vi "Fit Plots Cluster to Array.vi"(0 "Fit Plots in":T2, 1 "Plot Interpolation":T1=enum."Line (-)", 2 "Decay Fit Plot Name":string, 3 "Color Array in":u32[](array[colorbox])) -> (5 "Residuals Plot?":bool, 6 "Fit Plot Array":cluster{"t Array":dbl[], "Fitted Array":dbl[]}[](array[cluster]), 7 "Plot Names":string[](array[string]), 8 "CI Plots?":bool, 9 "Color Array out":u32[](array[colorbox]))   [LabVIEW 2021, in "AlliGator Decay Fit.lvlib"]
uses:
  AlliGator/Decay Analysis/Decay Fit/AlliGator Decay Fit.lvlib
  Fit Plots.ctl
  Graphs/LabVIEW Plot Interpolation.ctl
  Graphs/XY Graph/XY Graph Add-Ons.lvlib
  Graphs/Graphs.lvlib
  Fits.lvlib
panel:
  # "see the License on the block diagram (Ctrl+E or Window:Show Block Diagram)"
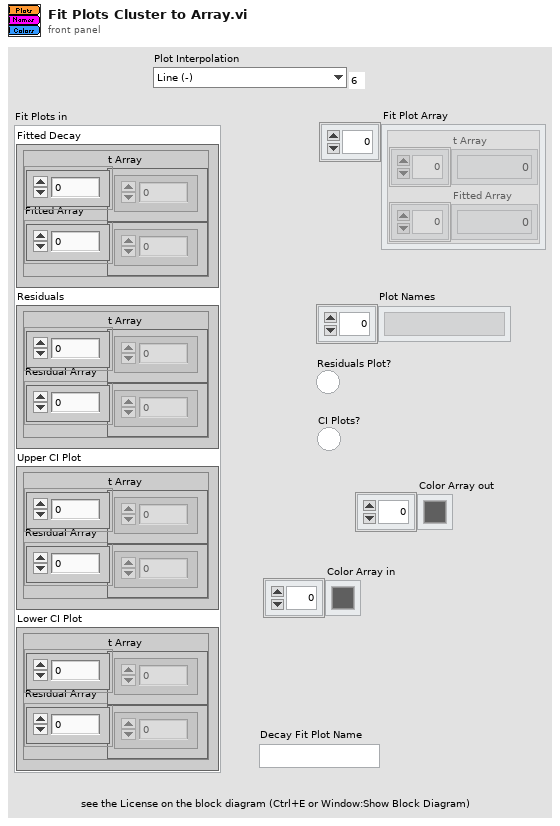
[diagram p1: front panel]
types:
  T1 = typedef "Graphs.lvlib/LabVIEW Plot Interpolation.ctl" = enum16{"Point (.)", "Stepwise Right (--.)", "Line + Point (\\. /)", "Stepwise Left (.--)", "Stepwise Centered (-.-)", "Stepwise Vertical (|.|)", "Line (-)", "Use Previous Plot's Style"}
  T2 = typedef "Fits.lvlib/Fit Plots.ctl" = cluster{"Fitted Decay":cluster{"t Array":dbl[], "Fitted Array":dbl[]}, "Residuals":cluster{"t Array":dbl[], "Residual Array":dbl[]}, "Upper CI Plot":cluster{"t Array":dbl[], "Residual Array":dbl[]}, "Lower CI Plot":cluster{"t Array":dbl[], "Residual Array":dbl[]}}
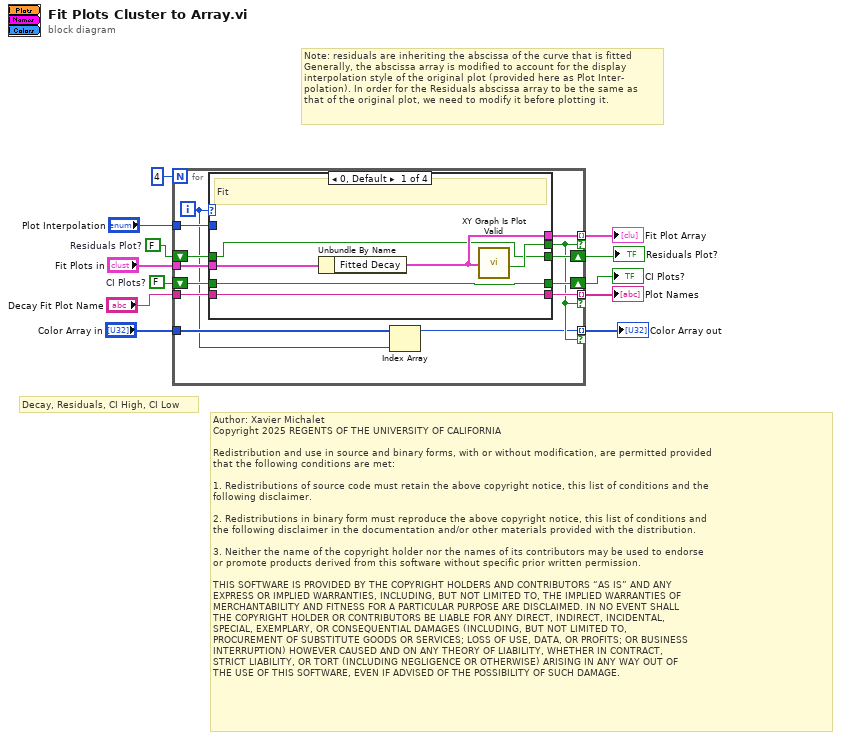
[diagram p0: block diagram]
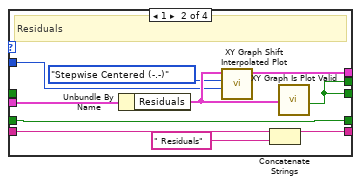
[diagram p2: hidden frame]
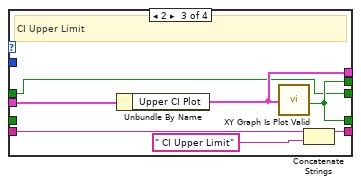
[diagram p3: hidden frame]
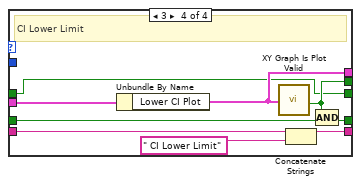
[diagram p4: hidden frame]
diagram:
  w3 = FALSE  # Residuals Plot?
  w7 = FALSE  # CI Plots?
  # "Decay, Residuals, CI High, CI Low"
  # "Note: residuals are inheriting the abscissa of the curve that is fitted\nGenerally, the abscissa array is modified to account for the display\ninterpolation style of the original plot (provided here as Plot Inter-\npolation). In order for the Residuals abscissa array to be the same as\nthat of the original plot, we need to modify it before plotting it."
  # "Author: Xavier Michalet\nCopyright 2025 REGENTS OF THE UNIVERSITY OF CALIFORNIA\n\nRedistribution and use in source and binary forms, with or without modification, are permitted provided\nthat the following conditions are met:\n\n1. Redistributions of source code must retain the above copyright notice, this list of conditions and the\nfollowing disclaimer.\n\n2. Redistributions in binary form must reproduce the above copyright notice, this list of conditions and\nthe following disclaimer in the documentation and/or other materials provided with the distribution.\n\n3. Neither the name of the copyright holder nor the names of its contributors may be used to endorse \nor promote products derived from this software without specific prior written permission.\n\nTHIS SOFTWARE IS PROVIDED BY THE COPYRIGHT HOLDERS AND CONTRIBUTORS “AS IS” AND ANY \nEXPRESS OR IMPLIED WARRANTIES, INCLUDING, BUT NOT LIMITED TO, THE IMPLIED WARRANTIES OF\nMERCHANTABILITY AND FITNESS FOR A PARTICULAR PURPOSE ARE DISCLAIMED. IN NO EVENT SHALL\nTHE COPYRIGHT HOLDER OR CONTRIBUTORS BE LIABLE FOR ANY DIRECT, INDIRECT, INCIDENTAL, \nSPECIAL, EXEMPLARY, OR CONSEQUENTIAL DAMAGES (INCLUDING, BUT NOT LIMITED TO, \nPROCUREMENT OF SUBSTITUTE GOODS OR SERVICES; LOSS OF USE, DATA, OR PROFITS; OR BUSINESS\nINTERRUPTION) HOWEVER CAUSED AND ON ANY THEORY OF LIABILITY, WHETHER IN CONTRACT, \nSTRICT LIABILITY, OR TORT (INCLUDING NEGLIGENCE OR OTHERWISE) ARISING IN ANY WAY OUT OF\nTHE USE OF THIS SOFTWARE, EVEN IF ADVISED OF THE POSSIBILITY OF SUCH DAMAGE."
  n1 = for {
    N: 4 -> [_]
    tunnel: "Fit Plots in" -> [w25]
    tunnel: [w24] -> w10 mode=indexing if=w16
    tunnel: "Decay Fit Plot Name" -> [w23]
    tunnel: [w22] -> w8 mode=indexing if=w16
    shift-right: [w21] -> w6
    shift-left: w7 -> [w20]
    tunnel: "Plot Interpolation" -> [w19]
    shift-right: [w18] -> w4
    shift-left: w3 -> [w17]
    tunnel: "Color Array in" -> [w15]
    tunnel: [w13] -> w1 mode=indexing if=w16
    i -> [w14]
    n2 = case shown="0, Default" w14 {
      tunnel: w25 -> [w31 w41 w48 w57]
      tunnel: [w30 w36 w47 w56] -> w24
      tunnel: [w29 w32 w43 w52] -> w16
      tunnel: w23 -> [w28 w40 w45 w55]
      tunnel: [w28 w38 w44 w54] -> w22
      tunnel: [w27 w37 w43 w50] -> w21
      tunnel: w20 -> [w27 w37 _ w51]
      tunnel: w19 -> [_ w34 _ _]
      tunnel: [w26 w32 w42 w49] -> w18
      tunnel: w17 -> [w26 _ w42 w49]
      frame 0, Default {
        # "Fit"
        n3 = Unbundle By Name(w31) -> ("Fitted Decay"=w30:cluster{"t Array":dbl[], "Fitted Array":dbl[]})
        n4 = call "XY Graph Is Plot Valid.vi"("Plot"=w30) -> ("Is Valid Plot?"=w29:bool)  [unwired: 8 in]
      }
      frame 1 {
        # "Residuals"
        n5 = Unbundle By Name(w41) -> ("Residuals"=w35:cluster{"t Array":dbl[], "Residual Array":dbl[]})
        n6 = call "XY Graph Shift Interpolated Plot.vi"("Plot Interpolation (out)"=w34, "Plot Interpolation (in)"=LabVIEW_Plot_Interpolation."Stepwise Centered (-.-)", "Plot in"=w35) -> ("Plot out"=w36:cluster{"t Array":dbl[], "Residual Array":dbl[]})  [unwired: 7 in, 1 out]
        n7 = Concatenate Strings(w40, " Residuals" ("string")) -> (w38:string)
        n8 = call "XY Graph Is Plot Valid.vi"("Plot"=w35) -> ("Is Valid Plot?"=w32:bool)  [unwired: 8 in]
      }
      frame 2 {
        # "CI Upper Limit"
        n9 = Unbundle By Name(w48) -> ("Upper CI Plot"=w47:cluster{"t Array":dbl[], "Residual Array":dbl[]})
        n10 = call "XY Graph Is Plot Valid.vi"("Plot"=w47) -> ("Is Valid Plot?"=w43:bool)  [unwired: 8 in]
        n11 = Concatenate Strings(w45, " CI Upper Limit" ("string")) -> (w44:string)
      }
      frame 3 {
        # "CI Lower Limit"
        n12 = Unbundle By Name(w57) -> ("Lower CI Plot"=w56:cluster{"t Array":dbl[], "Residual Array":dbl[]})
        n13 = call "XY Graph Is Plot Valid.vi"("Plot"=w56) -> ("Is Valid Plot?"=w52:bool)  [unwired: 8 in]
        n14 = Concatenate Strings(w55, " CI Lower Limit" ("string")) -> (w54:string)
        n15 = Compound Arithmetic op=AND(w52, w51) -> (w50:bool)
      }
    }
    n16 = Index Array(array=w15, index=w14) -> (element=w13:u32)
  }
  "Fit Plot Array" <- w10
  "Plot Names" <- w8
  "CI Plots?" <- w6
  "Residuals Plot?" <- w4
  "Color Array out" <- w1
